vi "Elevate Selection to Lowest Common Diagram.vi"(8 "error in":errorcluster, 11 "Selection in":refnum<vi>[](array[refnum])) -> (0 "error out":errorcluster, 2 "Lowest Common Diagram":refnum<vi>, 3 "Selection out":refnum<vi>[](array[refnum]))   [LabVIEW 2020, in "Enclose in Structure.lvlib"]
uses:
  Enclose in Structure.lvlib
  <vilib>/Utility/miscctls.llb/LVMapReplaceAction.ctl
  Selection Map.ctl
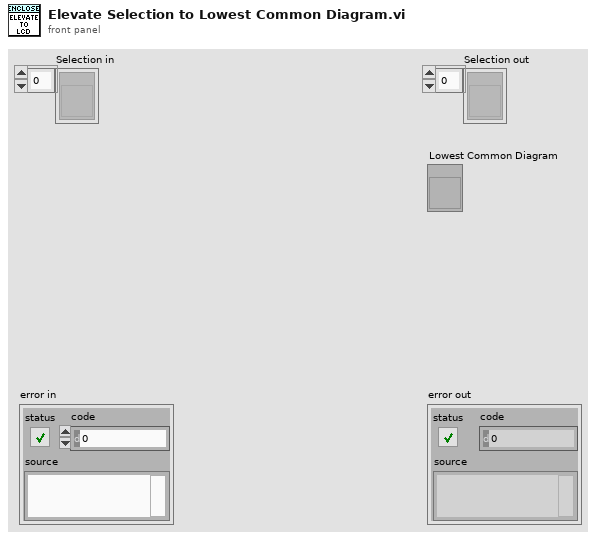
[diagram p1: front panel]
types:
  T1 = typedef "Enclose in Structure.lvlib/Selection Map.ctl" = map{i32, cluster{"Diag Ref":refnum<vi>, "Is Merge Point?":bool, "Selection":map{i32, refnum<vi>}, "Owning Diag UID":i32}}
  T2 = typedef "LVMapReplaceAction.ctl" = enum32{"Modify Entry only if found", "Add or Modify Entry", "Delete Entry"}
  T3 = cluster{"Diag Ref":refnum<vi>, "Is Merge Point?":bool, "Selection":map{i32, refnum<vi>}, "Owning Diag UID":i32}
  T4 = cluster{"Diag Ref":refnum<vi>, "Common":bool, "Selection":map{i32, refnum<vi>}, "Parent Diag UID":i32}
  T5 = cluster{"Diag Ref":refnum<vi>, "Common":bool, "Selection":map{i32, refnum<vi>}, "Owning Diag UID":i32}
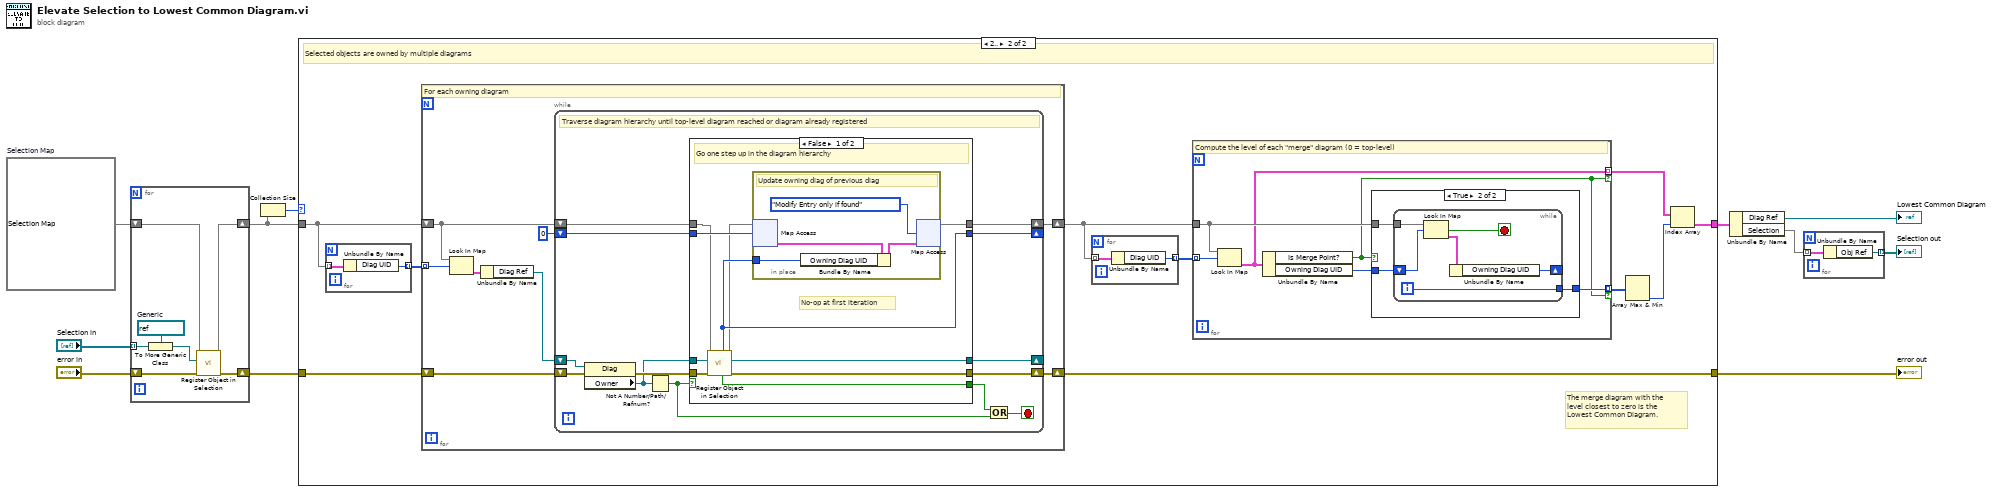
[diagram p0: block diagram]
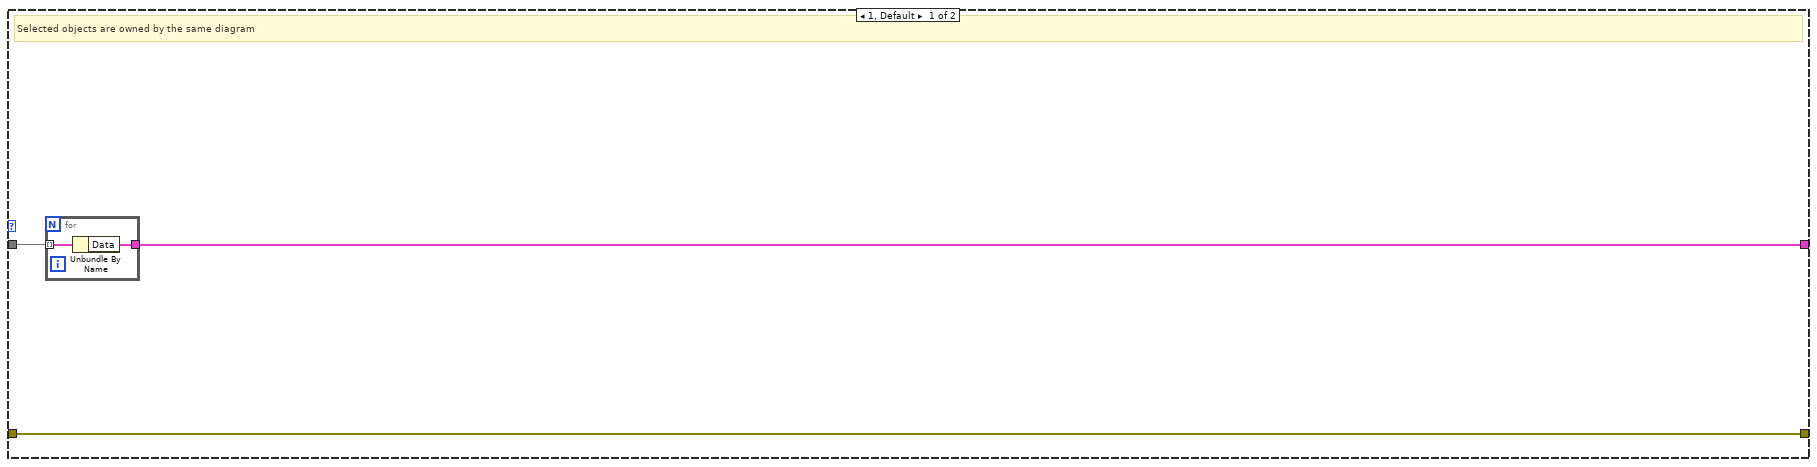
[diagram p2: hidden frame]
diagram:
  w1 = T1 {}  # Selection Map
  n1 = for {
    tunnel: "Selection in" -> [w15] mode=indexing
    shift-right: [w16] -> w9
    shift-left: w1 -> [w17]
    shift-right: [w12] -> w8
    shift-left: "error in" -> [w18]
    w13 = refnum<vi> refnum  # Generic
    n2 = To More Generic Class(target class=w13, reference=w15) -> (generic class reference=w14:refnum<vi>)
    n3 = call "Register Object in Selection.vi"("error in"=w18, "Object"=w14, "Selection in"=w17) -> ("error out"=w12:errorcluster, "Selection out"=w16:T1)  [unwired: 4 in, 3 out]
  }
  n4 = Collection Size(1:w9) -> (0:w6:i32)
  n5 = case shown="2.." w6 {
    tunnel: w9 -> [w20 w33]
    tunnel: w8 -> [w21 w31]
    tunnel: [w21 w30] -> w7
    tunnel: [w19 w25] -> w2
    frame 1, Default {
      # "Selected objects are owned by the same diagram"
      n6 = for {
        tunnel: w20 -> [w23] mode=indexing
        tunnel: [w22] -> w19
        n7 = Unbundle By Name(w23) -> ("Data"=w22:T3)
      }
    }
    frame 2.. {
      # "The merge diagram with the level closest to zero is the Lowest Common Diagram."
      # "Selected objects are owned by multiple diagrams"
      n8 = for {
        tunnel: w33 -> [w72] mode=indexing
        tunnel: [w71] -> w32 mode=indexing
        n9 = Unbundle By Name(w72) -> ("Diag UID"=w71:i32)
      }
      n10 = for {
        shift-right: [w35] -> w28
        shift-left: w33 -> [w36]
        tunnel: w32 -> [w41] mode=indexing
        shift-right: [w39] -> w30
        shift-left: w31 -> [w38]
        # "For each owning diagram"
        n11 = Look In Map(map=w36, key=w41) -> (value=w40:T4)  [unwired: 1 in, 1 out]
        n12 = Unbundle By Name(w40) -> ("Diag Ref"=w37:refnum<vi>)
        n13 = while {
          shift-right: [w48] -> w39
          shift-left: w38 -> [w54]
          shift-right: [w47] -> _
          shift-left: w37 -> [w52]
          shift-right: [w49] -> w35
          shift-left: w36 -> [w50]
          shift-right: [w43] -> _
          shift-left: 0 ("UID") -> [w42]
          stop <- w45 stop-if-true
          # "Traverse diagram hierarchy until top-level diagram reached or diagram already registered"
          n14 = property class="Diag"(reference=w52, error in=w54) -> (error out=w53:errorcluster, "Owner"=w51:refnum<vi>)  [unwired: 1 out]
          n15 = Not A Number/Path/Refnum?(number/path/refnum=w51) -> (NaN/Path/Refnum?=w46:bool)
          n16 = case shown="False" w46 {
            tunnel: w53 -> [w63 w70]
            tunnel: [w59 _] -> w47
            tunnel: w51 -> [w62 _]
            tunnel: w50 -> [w56 w69]
            tunnel: [w58 w69] -> w49
            tunnel: [w61 w70] -> w48
            tunnel: [w60 _] -> w44
            tunnel: [w57 _] -> w43
            tunnel: w42 -> [w64 _]
            frame False {
              # "No-op at first iteration"
              # "Go one step up in the diagram hierarchy"
              n17 = call "Register Object in Selection.vi"("error in"=w63, "Object"=w62, "Selection in"=w56) -> ("error out"=w61:errorcluster, "Owning Diag Ref"=w59:refnum<vi>, "Selection out"=w55:T1, "Owning Diag Already Registered?"=w60:bool, "Owning Diag UID"=w57:i32)  [unwired: 4 in]
              n18 = in-place {
                in-place-border: w57 -> [w66]
                # "Update owning diag of previous diag"
                n19 = in-place-map #1(w55, w64) -> (w68:T3)  [unwired: 1 in, 1 out]
                n20 = Bundle By Name(cluster=w68, "Owning Diag UID"=w66) -> (w67:T3)
                n21 = in-place-map #1(w67, LVMapReplaceAction."Modify Entry only if found" ("action")) -> (w58:T1)  [unwired: 2 out]
              }
            }
            frame True {
              # "Top-level diagram reached"
            }
          }
          n22 = Or(x=w44, y=w46) -> (x .or. y?=w45:bool)
        }
      }
      n23 = for {
        tunnel: w28 -> [w74] mode=indexing
        tunnel: [w73] -> w29 mode=indexing
        n24 = Unbundle By Name(w74) -> ("Diag UID"=w73:i32)
      }
      n25 = for {
        tunnel: w29 -> [w78] mode=indexing
        tunnel: w28 -> [w77]
        tunnel: [w76] -> w24 mode=indexing if=w75
        tunnel: [w79] -> w27 mode=indexing if=w75
        # "Compute the level of each \"merge\" diagram (0 = top-level)"
        n26 = Look In Map(map=w77, key=w78) -> (value=w76:T3)  [unwired: 1 in, 1 out]
        n27 = Unbundle By Name(w76) -> ("Is Merge Point?"=w75:bool, "Owning Diag UID"=w80:i32)
        n28 = case shown="True" w75 {
          tunnel: w80 -> [_ w83]
          tunnel: w77 -> [_ w82]
          tunnel: [_ w81] -> w79
          frame False {
          }
          frame True {
            n29 = while {
              tunnel: w82 -> [w89]
              shift-right: [w85] -> _
              shift-left: w83 -> [w88]
              tunnel: [w84] -> w81
              i -> [w84]
              stop <- w87 stop-if-true
              n30 = Look In Map(map=w89, key=w88) -> (key not found?=w87:bool, value=w86:T5)  [unwired: 1 in]
              n31 = Unbundle By Name(w86) -> ("Owning Diag UID"=w85:i32)
            }
          }
        }
      }
      n32 = Array Max & Min(array=w27) -> (min index (indices)=w26:i32)  [unwired: 3 out]
      n33 = Index Array(array=w24, index=w26) -> (element=w25:T3)
    }
  }
  "error out" <- w7
  n34 = Unbundle By Name(w2) -> ("Diag Ref"=→"Lowest Common Diagram":refnum<vi>, "Selection"=w5:map{i32, refnum<vi>})
  n35 = for {
    tunnel: w5 -> [w91] mode=indexing
    tunnel: [w90] -> w3 mode=indexing
    n36 = Unbundle By Name(w91) -> ("Obj Ref"=w90:refnum<vi>)
  }
  "Selection out" <- w3
